vi "From JSON.vi"(7 "LVClass Serializer":refnum<class "JSONtext LVClass Serializer.lvclass">, 8 "error in (no error)":errorcluster, 10 "<JSON>":string, 11 "Recursive JSON Serializable in":refnum<class "Recursive JSON Serializable.lvclass">) -> (0 "error out":errorcluster, 3 "Recursive JSON Serializable out":refnum<class "Recursive JSON Serializable.lvclass">)   [LabVIEW 2017, in "JSON Serializable Serializer Tests.lvlib" / "Recursive JSON Serializable.lvclass"]
doc: "Reads data from a JSON string."
uses:
  Recursive JSON Serializable.lvclass
  <vilib>/JDP Science/JSONtext/LVClass Serializer/JSONtext LVClass Serializer.lvclass
  Recursive JSON Serializable.lvclass/Recursive JSON Serializable.ctl
  <vilib>/JDP Science/JSONtext/JSONtext.lvlib
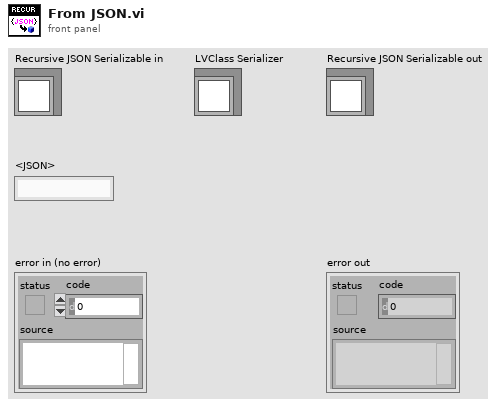
[diagram p1: front panel]
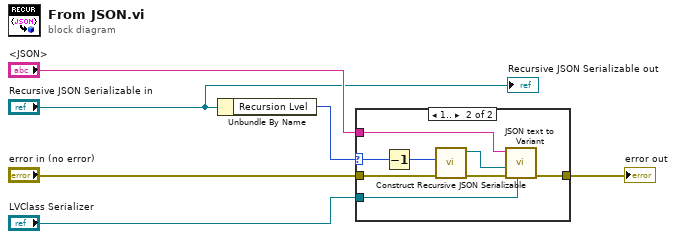
[diagram p0: block diagram]
diagram:
  n1 = Unbundle By Name("Recursive JSON Serializable in") -> ("Recursion Lvel"=w1:u8)
  n2 = case shown="1.." w1 {
    selector: w1 -> [_ w10]
    tunnel: [w7 w15] -> w6
    tunnel: "error in (no error)" -> [w7 w14]
    tunnel: "LVClass Serializer" -> [_ w13]
    tunnel: "<JSON>" -> [_ w12]
    frame 0 {
    }
    frame 1.. {
      n3 = Decrement(x=w10) -> (x-1=w9:u8)
      n4 = call "Construct Recursive JSON Serializable.vi"("error in (no error)"=w14, "Recursion Level"=w9) -> ("error out"=w11:errorcluster, "Recursive JSON Serializable"=w8:refnum<class "Recursive JSON Serializable.lvclass">)  [unwired: 8 in]
      n5 = call <vilib>:"JSON text to Variant.vi"("LVClass Serializer"=w13, "error in (no error)"=w11, "Data Type"=w8, "JSON"=w12) -> ("error out"=w15:errorcluster)  [unwired: 6 in, 1 out]
    }
  }
  "error out" <- w6
  "Recursive JSON Serializable out" <- "Recursive JSON Serializable in"
